vi "WaitMsecs.vi"(8 "error in (no error)":errorcluster, 9 "Title Message":string="Waiting countdown bar", 10 "Show progress bar?":bool, 11 "Wait Msecs":u32) -> (0 "error out":errorcluster)   [LabVIEW 2024]
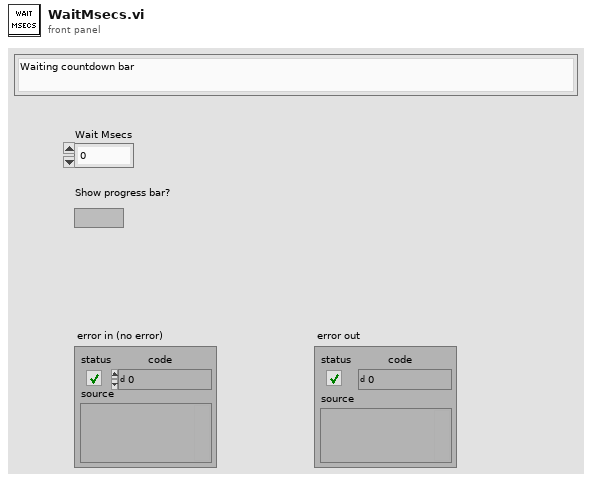
[diagram p1: front panel]
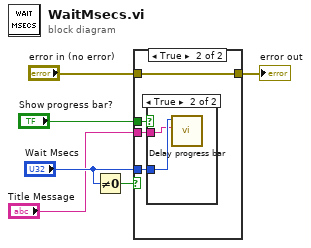
[diagram p0: block diagram]
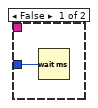
[diagram p3: hidden frame]
diagram:
  n1 = Not Equal To 0?(x="Wait Msecs") -> (x != 0?=w5:bool)
  n2 = case shown="True" w5 {
    tunnel: "Wait Msecs" -> [_ w11]
    tunnel: [w7 w10] -> w4
    tunnel: "error in (no error)" -> [w7 w10]
    tunnel: "Show progress bar?" -> [_ w9]
    tunnel: "Title Message" -> [_ w8]
    frame False {
    }
    frame True {
      n3 = case shown="True" w9 {
        tunnel: w11 -> [w12 w14]
        tunnel: w8 -> [_ w13]
        frame False {
          n4 = Wait (ms)(milliseconds to wait=w12) -> ()  [unwired: 1 out]
        }
        frame True {
          n5 = call "Delay progress bar.vi"("Title Message"=w13, "delay time mecs"=w14) -> ()  [unwired: 9 in, 1 out]
        }
      }
    }
  }
  "error out" <- w4
